vi "hidSPD Parse SPDClient JSON.vi"() -> ()   [LabVIEW 2018, in "hidSPDLibForLabView.lvlib"]
uses:
  hidSPDLibForLabView.lvlib
panel:
  out "Array":string[](array[string])
  out "error out":errorcluster
  out "text":string
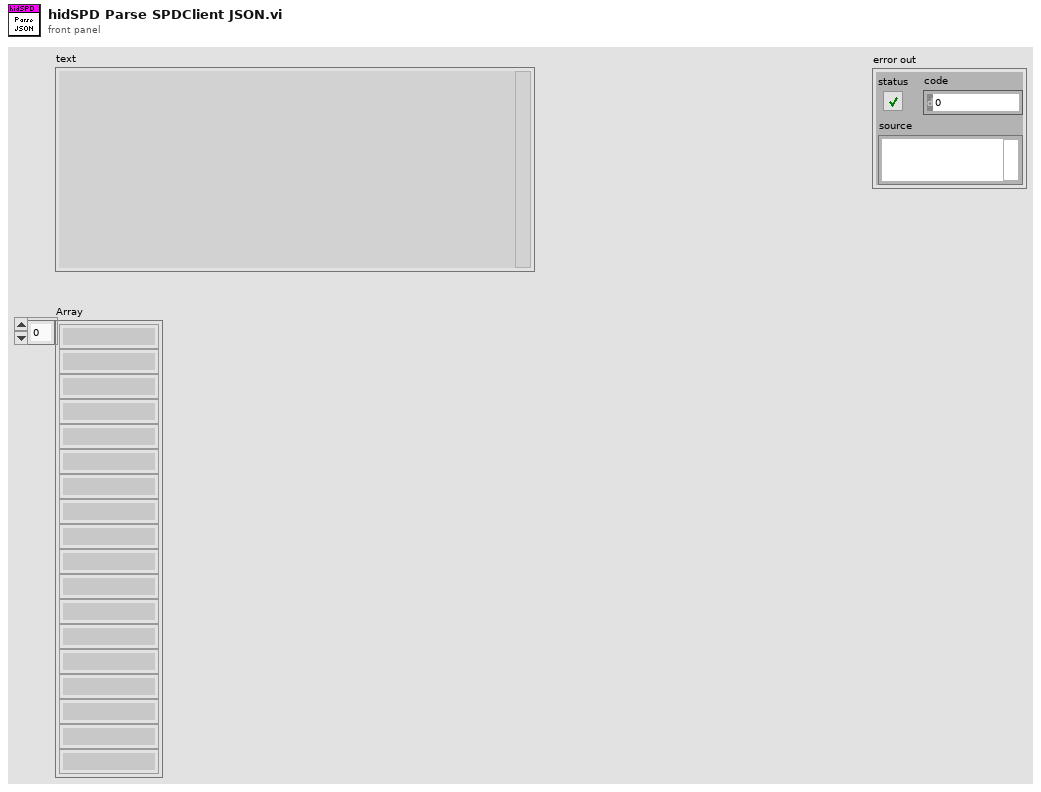
[diagram p1: front panel]
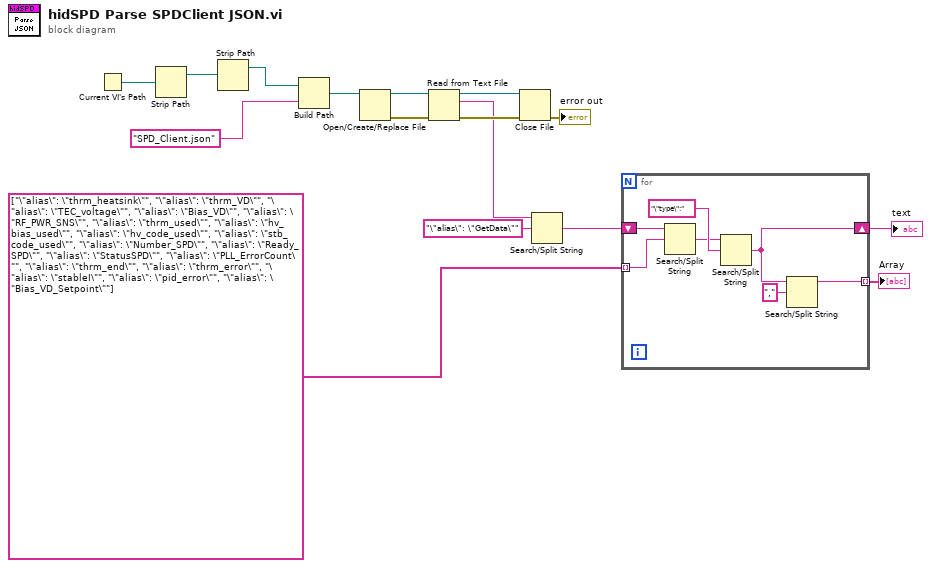
[diagram p0: block diagram]
diagram:
  n1 = Current VI's Path() -> (path=w16:path)
  n2 = Strip Path(path=w16) -> (stripped path=w15:path)  [unwired: 1 out]
  n3 = Strip Path(path=w15) -> (stripped path=w14:path)  [unwired: 1 out]
  n4 = Build Path(base path=w14, name or relative path="SPD_Client.json") -> (appended path=w12:path)
  n5 = Open/Create/Replace File(file path (use dialog)=w12) -> (refnum out=w11:refnum<file>, error out=w10:errorcluster)  [unwired: 5 in, 1 out]
  n6 = Read from Text File(file (use dialog)=w11, error in=w10) -> (refnum out=w9:refnum<file>, text=w6:string, error out=w8:errorcluster)  [unwired: 2 in, 1 out]
  n7 = Close File(refnum=w9, error in=w8) -> (error out=→"error out":errorcluster)  [unwired: 1 out]
  n8 = Search/Split String(string=w6, search string/char (-)="\"alias\": \"GetData\"") -> (match + rest of string=w4:string)  [unwired: 1 in, 2 out]
  n9 = for {
    shift-right: [w19] -> w2
    shift-left: w4 -> [w23]
    tunnel: string[] ["\"alias\": \"thrm_heatsink\"", "\"alias\": \"thrm_VD\"", "\"alias\": \"TEC_voltage\"", "\"alias\": \"Bias_VD\"", "\"alias\": \"RF_PWR_SNS\"", "\"alias\": \"thrm_used\"", "\"alias\": \"hv_bias_used\"", "\"alias\": \"hv_code_used\"", "\"alias\": \"stb_code_used\"", "\"alias\": \"Number_SPD\"", "\"alias\": \"Ready_SPD\"", "\"alias\": \"StatusSPD\"", "\"alias\": \"PLL_ErrorCount\"", "\"alias\": \"thrm_end\"", "\"alias\": \"thrm_error\"", "\"alias\": \"stableI\"", "\"alias\": \"pid_error\"", "\"alias\": \"Bias_VD_Setpoint\""] ("search string/char (-)") -> [w22] mode=indexing
    tunnel: [w17] -> w1 mode=indexing
    n10 = Search/Split String(string=w23, search string/char (-)=w22) -> (match + rest of string=w20:string)  [unwired: 1 in, 2 out]
    n11 = Search/Split String(string=w20, search string/char (-)="\"type\":") -> (match + rest of string=w19:string)  [unwired: 1 in, 2 out]
    n12 = Search/Split String(string=w19, search string/char (-)=",") -> (substring before match=w17:string)  [unwired: 1 in, 2 out]
  }
  "text" <- w2
  "Array" <- w1
